vi "Clear All Definitions in Disk.vi"(8 "error in (no error)":errorcluster, 11 "Bundle Builder in":refnum<class "Bundle Builder.lvclass">) -> (0 "error out":errorcluster, 3 "Bundle Builder out":refnum<class "Bundle Builder.lvclass">)   [LabVIEW 2020, in "Bundle Builder.lvclass"]
uses:
  Bundle Builder.lvclass
  Bundle Builder.lvclass/Bundle Builder.ctl
  <vilib>/Utility/error.llb/Error Cluster From Error Code.vi
  <vilib>/ErrorRing/Error Ring.xnode
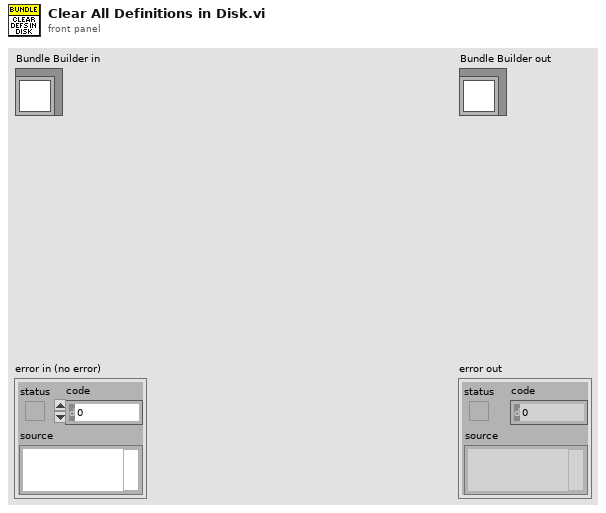
[diagram p1: front panel]
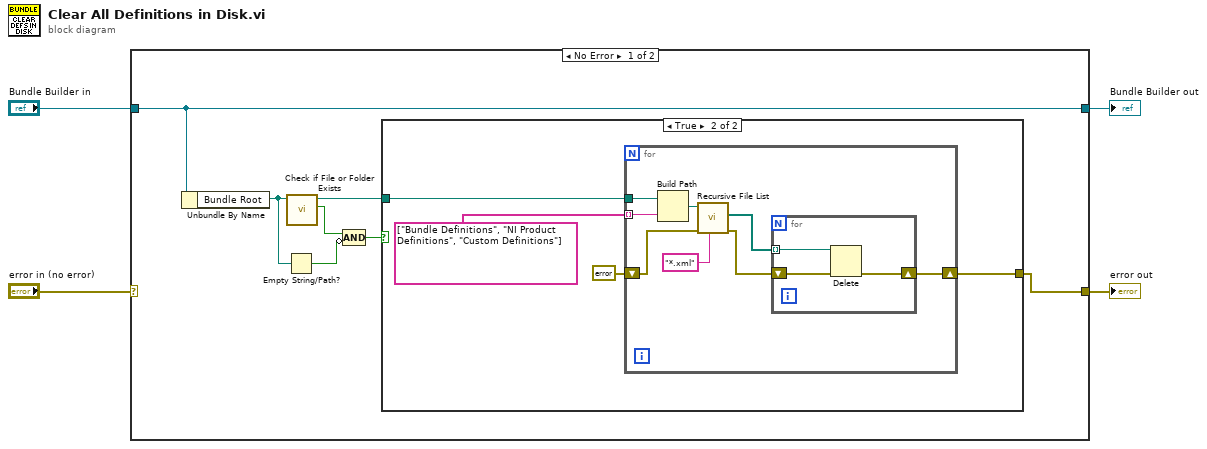
[diagram p0: block diagram]
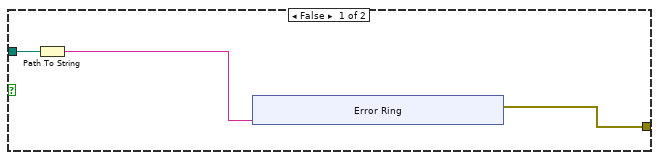
[diagram p2: hidden frame]
diagram:
  n1 = case shown="No Error" "error in (no error)" {
    selector: "error in (no error)" -> [_ w38]
    tunnel: [w5 w38] -> w3
    tunnel: [w11 w37] -> w1
    tunnel: "Bundle Builder in" -> [w11 w37]
    frame No Error {
      n2 = Unbundle By Name(w11) -> ("Bundle Root"=w10:path)
      n3 = Empty String/Path?(string/path=w10) -> (empty?=w8:bool)
      n4 = call <vilib>:"Check if File or Folder Exists.vi"("path"=w10) -> ("file or folder exists?"=w9:bool, "dup path"=w6:path)  [unwired: 8 in, 1 out]
      n5 = Compound Arithmetic op=AND(w9, invert w8) -> (w7:bool)
      n6 = case shown="True" w7 {
        tunnel: w6 -> [w14 w25]
        tunnel: [w12 w22] -> w5
        frame False {
          n7 = Path To String(path=w14) -> (string=w13:string)
          n8 = xnode "Error Ring"("parameter 0"=w13) -> ("error out"=w12:errorcluster)
        }
        frame True {
          n9 = for {
            tunnel: w25 -> [w33]
            tunnel: string[] ["Bundle Definitions", "NI Product Definitions", "Custom Definitions"] -> [w32] mode=indexing
            shift-right: [w27] -> w22
            shift-left: errorcluster {"status"=FALSE, "code"=0, "source"=""} ("error out") -> [w26]
            n10 = Build Path(base path=w33, name or relative path=w32) -> (appended path=w31:path)
            n11 = call <vilib>:"Recursive File List.vi"("pattern"="*.xml", "error in (no error)"=w26, "Folder Path"=w31) -> ("error out"=w28:errorcluster, "All Files in Dir"=w29:path[])  [unwired: 4 in, 3 out]
            n12 = for {
              tunnel: w29 -> [w36] mode=indexing
              shift-right: [w34] -> w27
              shift-left: w28 -> [w35]
              n13 = Delete(path (use dialog)=w36, error in=w35) -> (error out=w34:errorcluster)  [unwired: 3 in, 2 out]
            }
          }
        }
      }
    }
    frame Error {
    }
  }
  "error out" <- w3
  "Bundle Builder out" <- w1
